vi "PicoScope5000aGetValuesOverlappedBulk.vi"(5 "Segment Range":T1 {"toSegmentIndex" format="%.4p"; "fromSegmentIndex" format="%.4p"}, 7 "Buffer and Transfer Settings":T2={"startIndex"=0, "Samples"=1000, "Down Sample Ratio"=1, "Down-Sample Mode"=1} {"Down-Sample Mode" items=["None"=2147483648, "Aggregate"=1, "Decimate"=2, "Average"=4]; "Down Sample Ratio" step=1; "Samples" format="%_6p"}, 8 "error in (no error)":errorcluster, 11 "handle in":i16) -> (0 "error out":errorcluster, 3 "handle out":i16, 4 "overflow":i16[](array[numeric]) format="%010b", 6 "noOfSamples":u64)   [LabVIEW 2020]
doc: "Calls ps5000aGetValuesOverlappedBulk"
uses:
  Buffer and Transfer Settings.ctl
  Segment Range.ctl
  ps5000a.dll
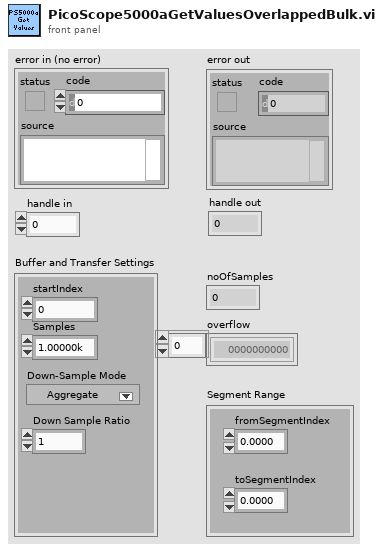
[diagram p1: front panel]
types:
  T1 = typedef "Segment Range.ctl" = cluster{"fromSegmentIndex":u64, "toSegmentIndex":u64}
  T2 = typedef "Buffer and Transfer Settings.ctl" = cluster{"startIndex":u64, "Samples":u64, "Down Sample Ratio":u64, "Down-Sample Mode":u32}
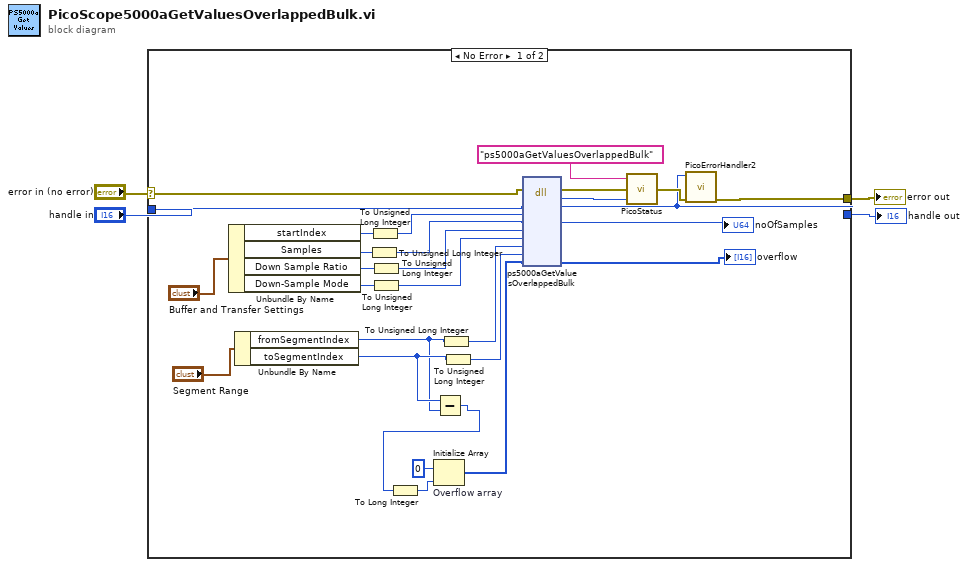
[diagram p0: block diagram]
diagram:
  n1 = case shown="No Error" "error in (no error)" {
    selector: "error in (no error)" -> [w19 w33]
    tunnel: "handle in" -> [w20 w34]
    tunnel: [w26 w34] -> w4
    tunnel: [w29 w33] -> w3
    frame No Error {
      n2 = Unbundle By Name("Buffer and Transfer Settings") -> ("startIndex"=w13:u64, "Samples"=w11:u64, "Down Sample Ratio"=w10:u64, "Down-Sample Mode"=w9:u32)
      n3 = Unbundle By Name("Segment Range") -> ("fromSegmentIndex"=w16:u64, "toSegmentIndex"=w17:u64)
      n4 = To Unsigned Long Integer(number=w11) -> (unsigned 32bit integer=w8:u32)
      n5 = To Unsigned Long Integer(number=w13) -> (unsigned 32bit integer=w12:u32)
      n6 = To Unsigned Long Integer(number=w10) -> (unsigned 32bit integer=w7:u32)
      n7 = To Unsigned Long Integer(number=w9) -> (unsigned 32bit integer=w6:u32)
      n8 = Subtract(x=w17, y=w16) -> (x-y=w21:u64)
      n9 = To Long Integer(number=w21) -> (32bit integer=w23:i32)
      n10 = Initialize Array "Overflow array"(i16 0 ("element"), w23) -> (w22:i16[])
      n11 = To Unsigned Long Integer(number=w16) -> (unsigned 32bit integer=w15:u32)
      n12 = To Unsigned Long Integer(number=w17) -> (unsigned 32bit integer=w14:u32)
      n13 = dll-call lib="ps5000a.dll" fn="ps5000aGetValuesOverlappedBulk" ("ps3000.dll:_ps3000_open_unit@0")(error in=w19, "handle"=w20, "startIndex"=w12, "noOfSamples"=w8, "downSampleRatio"=w7, "downSampleRatioMode"=w6, "fromSegmentIndex"=w15, "toSegmentIndex"=w14, "overflow"=w22) -> (error out=w27:errorcluster, "PICO_STATUS"=w25:u32, "handle"=w26:i16, "noOfSamples"=→"noOfSamples":u32, "overflow"=→"overflow":i16[])  [unwired: 7 in, 1 out]
      n14 = call "PicoStatus.vi"("PICO STATUS"=w25, "error in"=w27, "source"="ps5000aGetValuesOverlappedBulk") -> ("error out"=w32:errorcluster)
      n15 = call "PicoErrorHandler2.vi"("error in (no error)"=w32, "handle In"=w26) -> ("error out"=w29:errorcluster)  [unwired: 9 in]
    }
    frame Error {
    }
  }
  "error out" <- w3
  "handle out" <- w4
